vi "THz Time(SR830_VC_PSD_MCS)_TA_170401.vi"(4 "Lockin Address":string="12") -> ()   [LabVIEW 2010]
panel:
  in  "?":bool
  out "Current Round":i32=160
  out "Current Gap (um)":u32=100
  out "error out 2":errorcluster
  in  "Initial Gap (um)":u32=100
  in  "Number of Gap":u32=8
  in  "Number of Avg":u32=20
  in  "Gap Increase (um)":u32=25
  in  "Step Increase (um)":u32=1
  in  "error in (no error)":errorcluster
  in  "MCS System Locator":string="usb:id:1441320285"
  in  "CONEX-PSD9 Instrument Key 2":string="CONEX-PSD (A6ULD73M)"
  in  "Exit Program":bool
  out "Y position":dbl=-5.0 format="%#.3p"
  out "X position":dbl=-5.0 format="%#.3p"
  out "Power meter":dbl format="%#.3p"
  in  "Launch server?":bool
  in  "Authorize?":bool=TRUE
  out "error out":errorcluster
  out "Position 2":dbl[](array[numeric])=[2.395] format="%.6f"
  in  "error in":errorcluster
  out "Running":bool caption="Mercury_GCS_Configuration_Setup.vi is running"
  out "Conn. Axis":string[](array[string])=["1"]
  out "Identification":string="(c)2013 Physik Instrumente(PI) Karlsruhe, C-863.11,0,1.3.0.7"
  in  "SaveFile name":string="t"
  in  "Interdelay (ms)":dbl=10.0
  in  "pre delay (ms)":dbl=100.0
  out "Lock-in Y-Channel":dbl=-7.0941e-11 format="%#.3p"
  out "Lock-in X-Channel":dbl=5.62071e-10 format="%#.3p"
  out "THz Time-domain Signal Wave":cluster{"x-axis":sgl[], "y-axis":dbl[]}(graph)={"x-axis"=[3.4, 3.395, 3.39, 3.385, 3.38, 3.375, 3.3700001, 3.365, 3.3600001, 3.355, 3.3500001, 3.345, 3.3400002, 3.335, 3.3300002, 3.325, 3.3200002, 3.315, 3.3100002, 3.305, 3.3000002, 3.295, 3.2900002, 3.285, 3.2800002, 3.275, 3.27, 3.265, 3.26, 3.255, 3.25, 3.2450001, 3.24, 3.2350001, 3.23, 3.2250001, 3.22, 3.2150002, 3.21, 3.2050002, 3.2, 3.1950002, 3.19, 3.1850002, 3.18, 3.1750002, 3.17, 3.1650002, 3.16, 3.1550002, 3.15, 3.1450002, 3.14, 3.135, 3.13, 3.125, 3.1200001, 3.115, 3.1100001, 3.105, 3.1000001, 3.095, 3.0900002, 3.085, 3.0800002, 3.075, 3.0700002, 3.065, 3.0600002, 3.055, 3.0500002, 3.045, 3.0400002, 3.035, 3.0300002, 3.025, 3.0200002, 3.015, 3.01, 3.005, 3.0, 2.9950001, 2.99, 2.9850001, 2.98, 2.9750001, 2.97, 2.9650002, 2.96, 2.9550002, 2.95, 2.9450002, 2.94, 2.9350002, 2.93, 2.9250002, 2.92, 2.9150002, 2.91, 2.9050002, 2.9, 2.8950002, 2.89, 2.885, 2.88, 2.875, 2.8700001, 2.865, 2.8600001, 2.855, 2.8500001, 2.845, 2.8400002, 2.835, 2.8300002, 2.825, 2.8200002, 2.815, 2.8100002, 2.805, 2.8000002, 2.795, 2.7900002, 2.785, 2.7800002, 2.775, 2.7700002, 2.765, 2.7600002, 2.755, 2.75, 2.7450001, 2.74, 2.7350001, 2.73, 2.7250001, 2.72, 2.7150002, 2.71, 2.7050002, 2.7, 2.6950002, 2.69, 2.6850002, 2.68, 2.6750002, 2.67, 2.6650002, 2.66, 2.6550002, 2.65, 2.6450002, 2.64, 2.6350002, 2.63, 2.625, 2.6200001, 2.615, 2.6100001, 2.605, 2.6000001, 2.595, 2.5900002, 2.585, 2.5800002, 2.575, 2.5700002, 2.565, 2.5600002, 2.555, 2.5500002, 2.545, 2.5400002, 2.535, 2.5300002, 2.525, 2.5200002, 2.515, 2.5100002, 2.505, 2.5, 2.4950001, 2.49, 2.4850001, 2.48, 2.4750001, 2.47, 2.4650002, 2.46, 2.4550002, 2.45, 2.4450002, 2.44, 2.4350002, 2.43, 2.4250002, 2.42, 2.4150002, 2.41, 2.4050002, 2.4, 2.3950002], "y-axis"=array[202 elements]}
  in  "Autosave Directory for Long-term Average Scan":path=path "D:/Soon/140901_delay_test/2_VC_delay_ESP_-2.35/1_VC_delay"
  in  "OK Button":bool
  out "Data Type":string="outp ? 1"
  in  "Enum":enum16{"X", "Y", "Abs"}(ring)
  in  "SCAN":bool
  in  "Short term \nAverage#":i8=2
  in  "Step":sgl=0.005 min=0 max=10000 format="%.3f"
  in  "End Postion":sgl=2.4 min=-400 max=400 format="%#.3f"
  in  "Start Position":sgl=3.4 min=-400 max=400 format="%#.3f"
  # "THz Experiment"
  # "``"
  # "Input Data"
  # "Auto-offset"
  # "Point Avg"
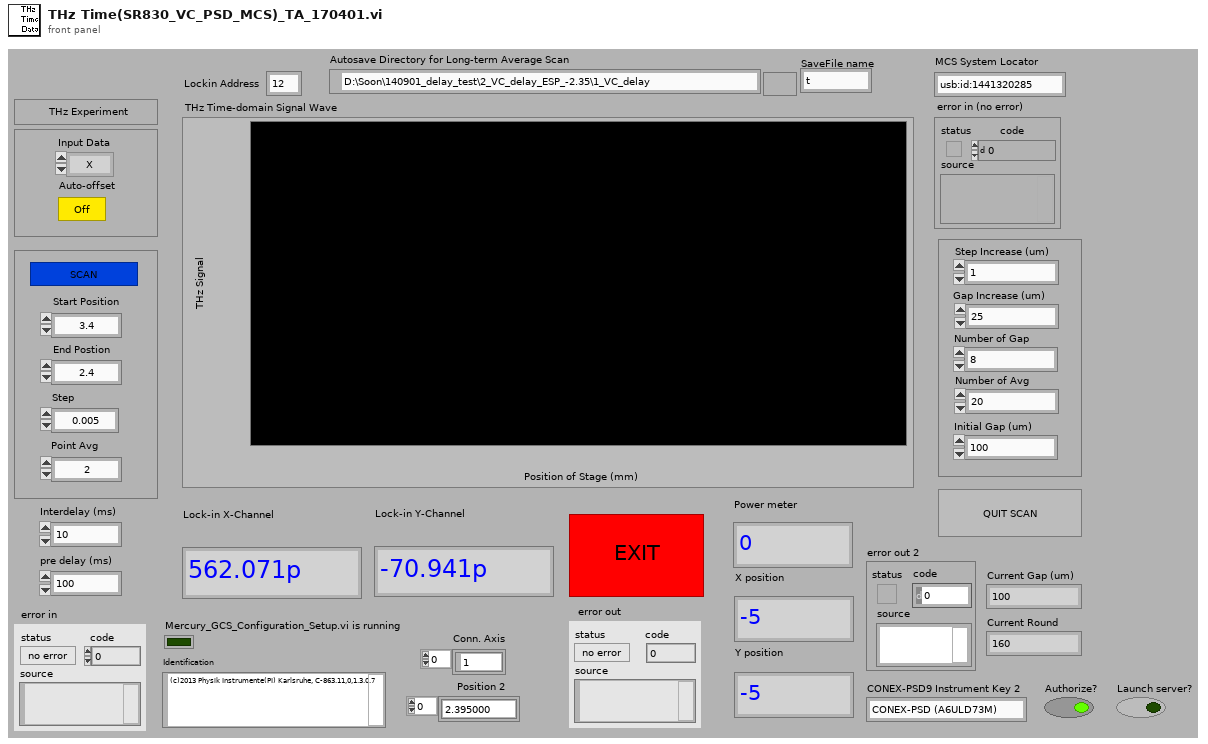
[diagram p1: front panel]
types:
  T1 = cluster{"System no.":i32, "error out":errorcluster}
  T2 = cluster{"ConexPSD Reference":refnum<k24>, "error out":errorcluster, "Component ID":i32}
  T3 = cluster{"System Index Out":u32, "error out":errorcluster}
  T4 = cluster{"Step Number":i32, "Step":sgl, "Start Position":sgl, "Time-out":i32, "Lockin Address":string, "Short term \nAverage#":i8, "System no.":i32, "error out":errorcluster, "Value":string, "pre delay (ms)":dbl, "Interdelay (ms)":dbl, "Autosave Directory for Long-term Average Scan":path, cluster{"ConexPSD Reference":refnum<k24>, "error out":errorcluster, "Component ID":i32}}
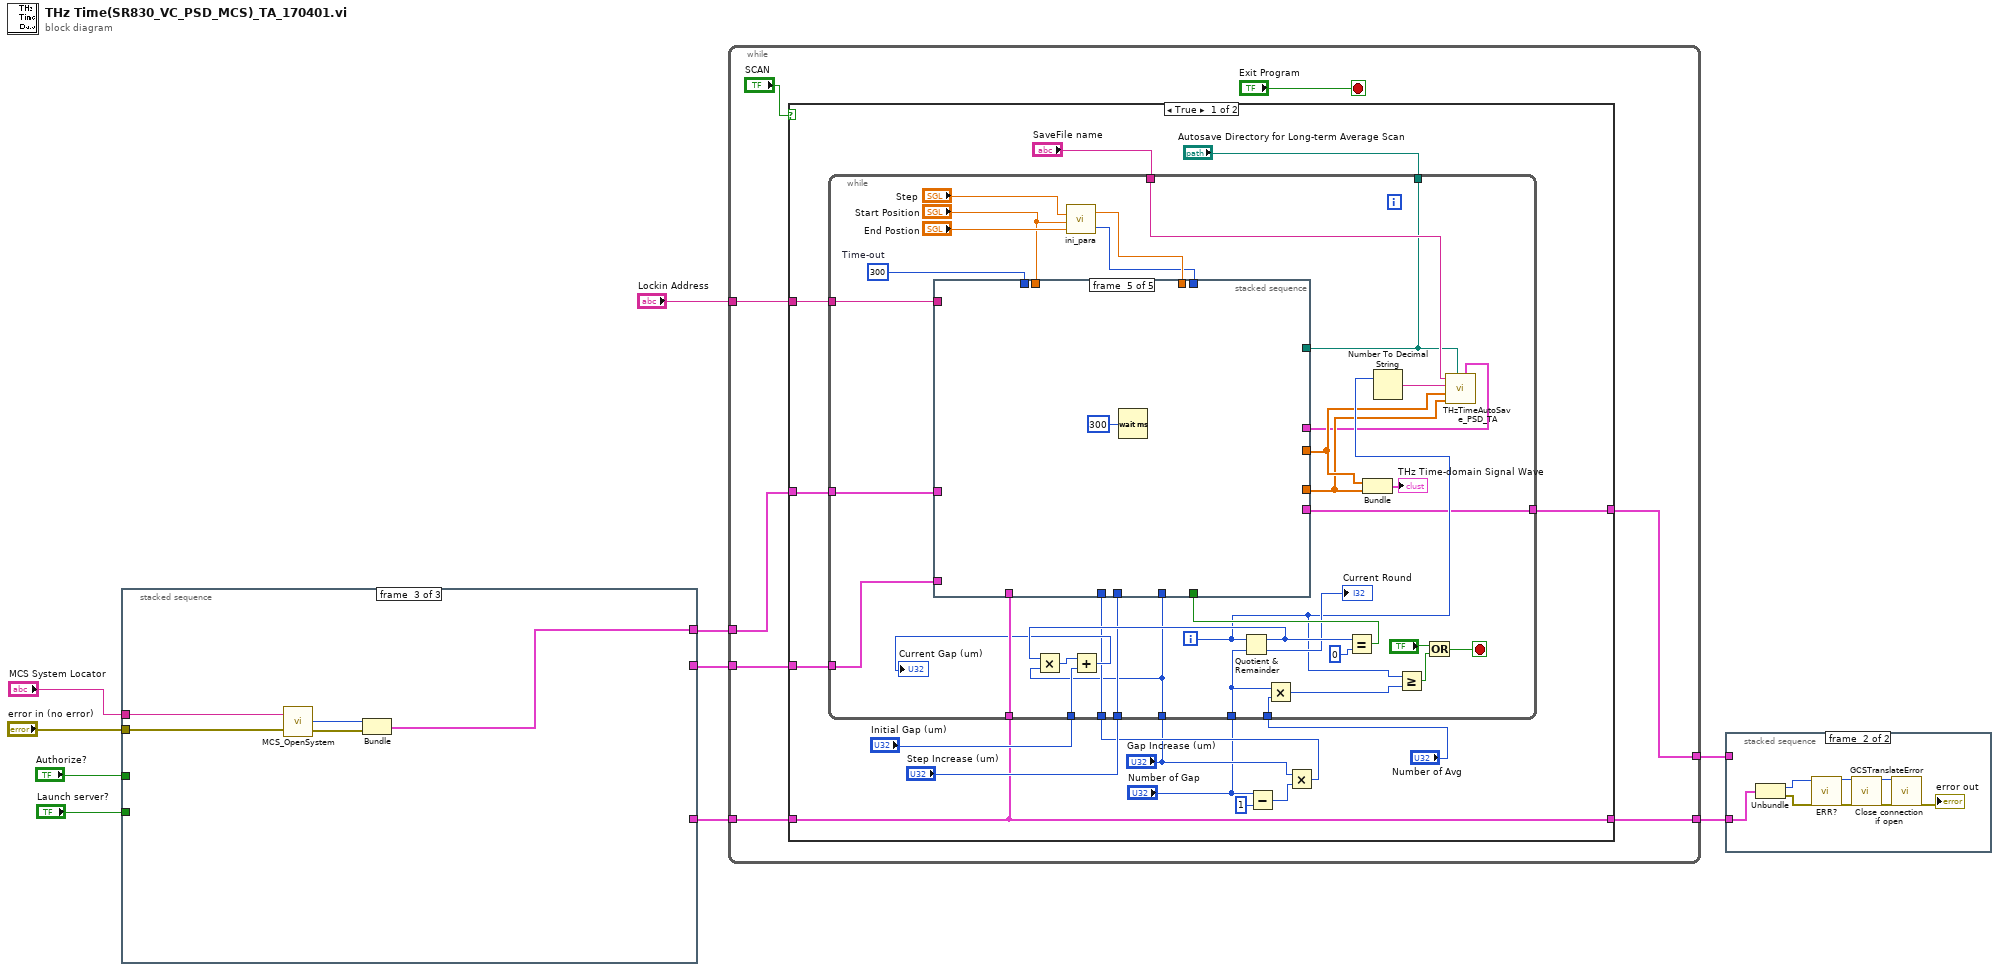
[diagram p0: block diagram]
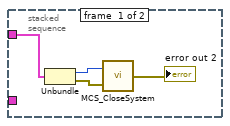
[diagram p2: hidden frame]
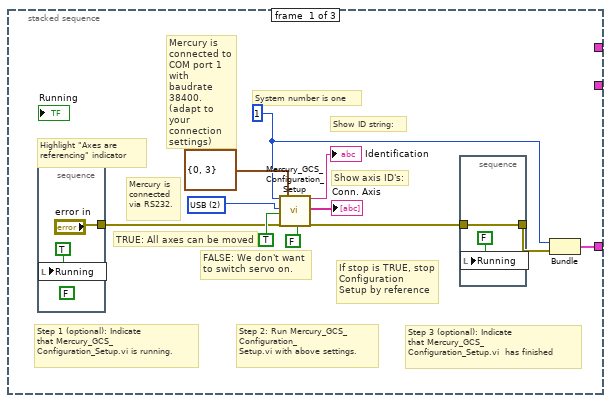
[diagram p3: hidden frame]
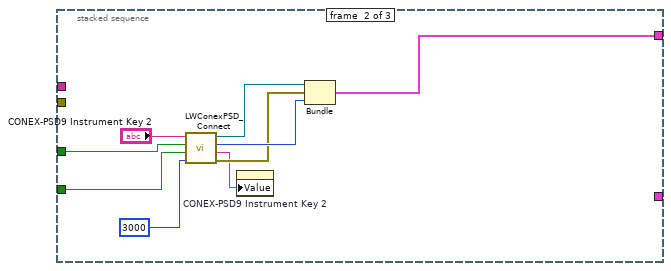
[diagram p4: hidden frame]
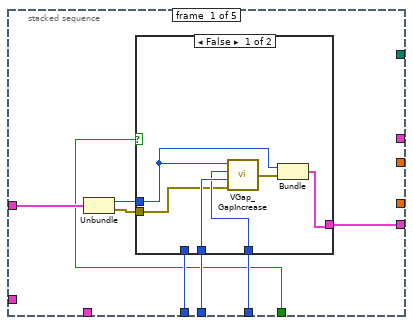
[diagram p5: hidden frame]
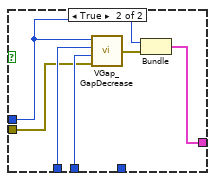
[diagram p6: hidden frame]
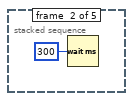
[diagram p7: hidden frame]
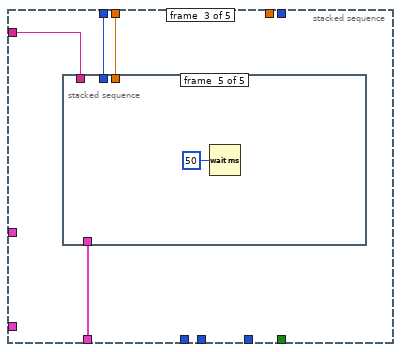
[diagram p8: hidden frame]
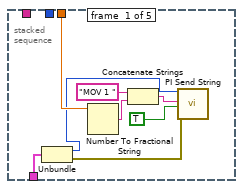
[diagram p9: hidden frame]
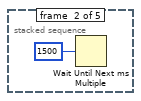
[diagram p10: hidden frame]
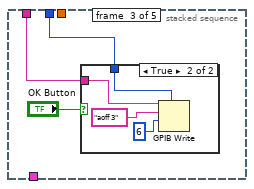
[diagram p11: hidden frame]
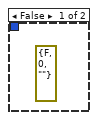
[diagram p12: hidden frame]
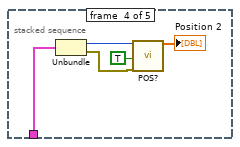
[diagram p13: hidden frame]
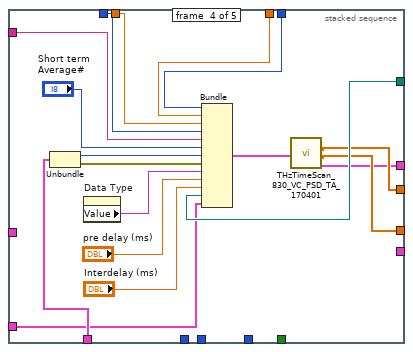
[diagram p14: hidden frame]
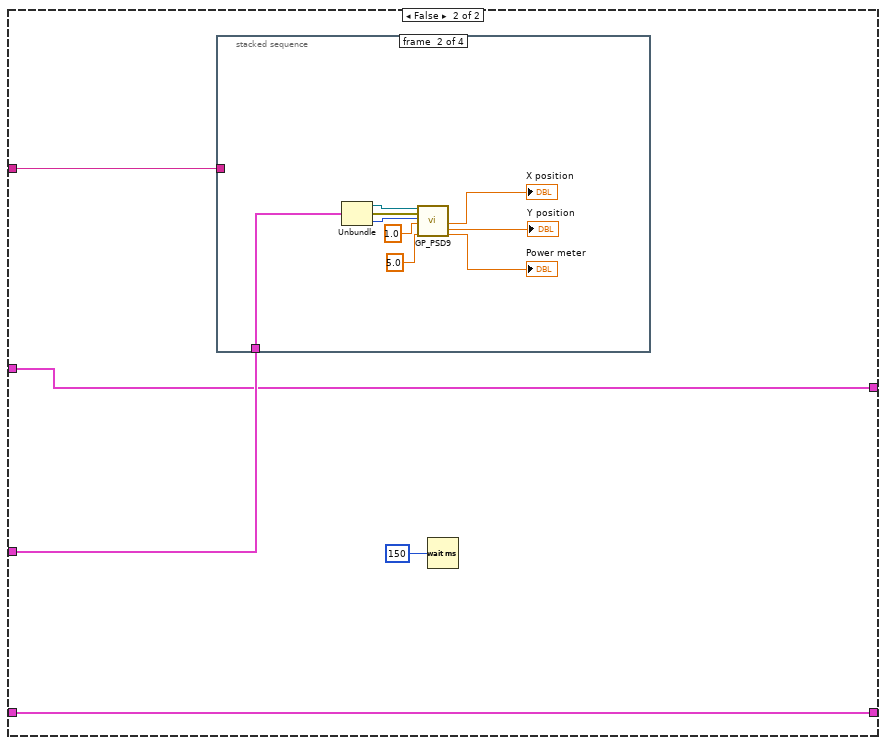
[diagram p15: hidden frame]
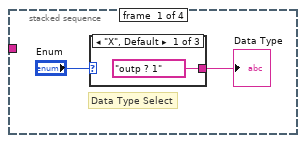
[diagram p16: hidden frame]
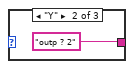
[diagram p17: hidden frame]
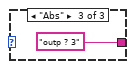
[diagram p18: hidden frame]
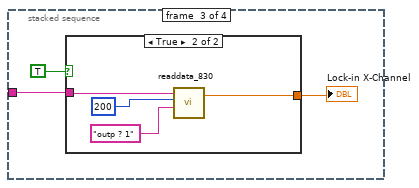
[diagram p19: hidden frame]
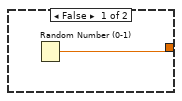
[diagram p20: hidden frame]
diagram:
  n1 = stacked-sequence {
    tunnel: "Authorize?" -> [_ w29 _]
    tunnel: "Launch server?" -> [_ w28 _]
    tunnel: [_ w26 _] -> w7
    tunnel: "MCS System Locator" -> [_ _ w37]
    tunnel: "error in (no error)" -> [_ _ w36]
    tunnel: [_ _ w35] -> w4
    tunnel: [w11 _ _] -> w3
    frame #0 {
      w14 = u16 2 items=["RS232", "RS232 DaisyChain", "USB", "USB_DaisyChain"] ("Interface")
      w12 = 1 ("System no.")
      # "Mercury is\nconnected\nvia RS232."
      # "If stop is TRUE, stop \nConfiguration\nSetup by reference"
      # "Mercury is\nconnected to\nCOM port 1\nwith baudrate\n38400.\n(adapt to your\nconnection\nsettings)"
      # "Step 3 (optional): Indicate\nthat Mercury_GCS_\nConfiguration_Setup.vi  has finished"
      # "Step 2: Run Mercury_GCS_\nConfiguration_\nSetup.vi with above settings."
      # "Step 1 (optional): Indicate\nthat Mercury_GCS_\nConfiguration_Setup.vi is running."
      # "Highlight \"Axes are\nreferencing\" indicator"
      # "Show axis ID's:"
      # "Show ID string:"
      # "FALSE: We don't want\nto switch servo on."
      # "TRUE: All axes can be moved"
      # "System number is one"
      n2 = stacked-sequence {
        tunnel: ["error in"] -> w17
        frame #0 {
          (unwired) FALSE ("stop")
          n3 = local write "Running"(TRUE ("Running")) -> ()
        }
      }
      n4 = call "Mercury_GCS_Configuration_Setup.vi"("System no."=w12, "Interface"=w14, "All axes?"=TRUE, "error in"=w17, "RS232 settings"=cluster{"RS232 Portnumber":i32, "Baudrate":u16} {"RS232 Portnumber"=0, "Baudrate"=3}, "Switch servo on?"=FALSE ("Use dialog to define\nconnected stages?")) -> ("Identification"=→"Identification":string, "Conn. \nAxes"=→"Conn. Axis":string[], "error out"=w18:errorcluster)  [unwired: 7 in, 4 out]
      n5 = stacked-sequence {
        tunnel: w18 -> [w25]
        tunnel: [w25] -> w13
        frame #0 {
          n6 = local write "Running"(FALSE ("Running")) -> ()
        }
      }
      n7 = Bundle("System no."=w12, "error out"=w13) -> (w11:T1)  [unwired: 1 in]
    }
    frame #1 {
      n8 = call "LWConexPSD_Connect.vi"("DiscoverTimeout (10000 msec)"=3000, "Launch server? (True)"=w28, "Authorize? (True)"=w29, "Instrument Key"="CONEX-PSD9 Instrument Key 2") -> ("error out"=w32:errorcluster, "Instrument Key out"=w31:string, "Component ID"=w33:i32, "ConexPSD Reference"=w27:refnum<k24>)
      n9 = property on="CONEX-PSD9 Instrument Key 2" class="Str"("Value"=w31) -> ()  [unwired: 2 in, 2 out]
      n10 = Bundle("ConexPSD Reference"=w27, "error out"=w32, "Component ID"=w33) -> (w26:T2)  [unwired: 1 in]
    }
    frame #2 {
      n11 = call "MCS_OpenSystem.vi"("error in (no error)"=w36, "MCS System Locator"=w37) -> ("error out"=w38:errorcluster, "System Index Out"=w39:u32)
      n12 = Bundle("System Index Out"=w39, "error out"=w38) -> (w35:T3)  [unwired: 1 in]
    }
  }
  n13 = while {
    tunnel: "Lockin Address" -> [w46]
    tunnel: w7 -> [w44]
    tunnel: w4 -> [w43]
    tunnel: w3 -> [w42]
    tunnel: [w41] -> w2
    tunnel: [w40] -> w1
    stop <- "Exit Program" stop-if-true
    n14 = case shown="True" "SCAN" {
      tunnel: w46 -> [w62 w167]
      tunnel: [w55 w165] -> w41
      tunnel: w44 -> [w49 w166]
      tunnel: w43 -> [w59 w164]
      tunnel: w42 -> [w55 w165]
      tunnel: [w48 w164] -> w40
      frame True {
        n15 = Subtract(x="Number of Gap", y=u32 1) -> (x-y=w53:u32)
        n16 = Multiply(x="Gap Increase (um)", y=w53) -> (x*y=w52:u32)
        n17 = while {
          tunnel: w62 -> [w97]
          tunnel: w55 -> [w96]
          tunnel: "SaveFile name" -> [w68]
          tunnel: "Autosave Directory for Long-term Average Scan" -> [w67]
          tunnel: w59 -> [w95]
          tunnel: "Initial Gap (um)" -> [w80]
          tunnel: "Step Increase (um)" -> [w77]
          tunnel: "Number of Avg" -> [w79]
          tunnel: w52 -> [w78]
          tunnel: "Gap Increase (um)" -> [w76]
          tunnel: "Number of Gap" -> [w75]
          tunnel: w49 -> [w66]
          tunnel: [w63] -> w48
          i -> [w71]
          stop <- w64 stop-if-true
          w94 = 300  # Time-out
          n18 = call "ini_para.vi"("End Position"="End Postion", "Start Position"="Start Position", "Step"="Step") -> ("Step Number"=w88:i32, "Step"=w89:sgl)
          n19 = Quotient & Remainder(x=w71, y=w75) -> (x-y*floor(x/y)=w86:u32, floor(x/y)=→"Current Round":u32)
          n20 = Multiply(x=w86, y=w76) -> (x*y=w85:u32)
          n21 = Add(x=w85, y=w80) -> (x+y=→"Current Gap (um)":u32)
          n22 = Multiply(x=w75, y=w79) -> (x*y=w82:u32)
          n23 = Equal?(x=w86, y=u32 0) -> (x = y?=w74:bool)
          n24 = stacked-sequence {
            tunnel: w94 -> [_ _ w122 w161 _]
            tunnel: "Start Position" -> [_ _ w121 w153 _]
            tunnel: w89 -> [_ _ _ w154 _]
            tunnel: w88 -> [_ _ _ w162 _]
            tunnel: [_ _ _ w146 _] -> w70
            tunnel: [_ _ _ w147 _] -> w69
            tunnel: w67 -> [_ _ _ w156 _]
            tunnel: w97 -> [_ _ w120 w155 _]
            tunnel: w96 -> [_ _ w119 w152 _]
            tunnel: w95 -> [w103 _ _ _ _]
            tunnel: w78 -> [w102 _ _ _ _]
            tunnel: w77 -> [w101 _ _ _ _]
            tunnel: w76 -> [w100 _ _ _ _]
            tunnel: w74 -> [w99 _ _ _ _]
            tunnel: w66 -> [_ _ _ w148 _]
            tunnel: [_ _ _ w145 _] -> w65
            tunnel: [w98 _ _ _ _] -> w63
            frame #0 {
              n25 = Unbundle(w103) -> ("System Index Out"=w104:u32, "error out"=w105:errorcluster)
              n26 = case shown="False" w99 {
                tunnel: w102 -> [_ w117]
                tunnel: w101 -> [w111 w116]
                tunnel: w100 -> [w110 _]
                tunnel: w104 -> [w107 w113]
                tunnel: w105 -> [w109 w115]
                tunnel: [w106 w112] -> w98
                frame False {
                  n27 = call "VGap_GapIncrease.vi"("error in (no error)"=w109, "Step Increase (um)"=w111, "Gap Increase (um)"=w110, "System Index In"=w107) -> ("error out"=w108:errorcluster)
                  n28 = Bundle("System Index Out"=w107, "error out"=w108) -> (w106:T3)  [unwired: 1 in]
                }
                frame True {
                  n29 = call "VGap_GapDecrease.vi"("error in (no error)"=w115, "Step Decrease (um)"=w116, "Gap Decrease (um)"=w117, "System Index In"=w113) -> ("error out"=w114:errorcluster)
                  n30 = Bundle("System Index Out"=w113, "error out"=w114) -> (w112:T3)  [unwired: 1 in]
                }
              }
            }
            frame #1 {
              n31 = Wait (ms)(milliseconds to wait=u32 300) -> ()  [unwired: 1 out]
            }
            frame #2 {
              n32 = stacked-sequence {
                tunnel: w122 -> [_ _ w133 _ _]
                tunnel: w121 -> [w126 _ _ _ _]
                tunnel: w120 -> [_ _ w132 _ _]
                tunnel: w119 -> [w125 _ _ w141 _]
                frame #0 {
                  n33 = Unbundle(w125) -> ("System no."=w123:i32, "error out"=w124:errorcluster)
                  n34 = Number To Fractional String(number=w126) -> (F-format string=w127:string)  [unwired: 3 in]
                  n35 = Concatenate Strings("MOV 1 ", w127) -> (w130:string)
                  n36 = call "PI Send String.vi"("System no."=w123, "String to send"=w130, "Attach termination char.?"=TRUE ("Attach Linefeed?"), "error in"=w124) -> ()  [unwired: 15 in, 1 out]
                }
                frame #1 {
                  n37 = Wait Until Next ms Multiple(millisecond multiple=1500) -> ()  [unwired: 1 out]
                }
                frame #2 {
                  n38 = case shown="True" "OK Button" {
                    tunnel: w133 -> [_ w137]
                    tunnel: w132 -> [_ w135]
                    frame False {
                      (unwired) errorcluster {"status"=FALSE, "code"=0, "source"=""} ("error in")
                    }
                    frame True {
                      n39 = GPIB Write(0:w135, 1:"aoff 3" ("data"), 2:i16 6 ("mode (0)"), 4:w137) -> ()  [unwired: 1 in, 2 out]
                    }
                  }
                }
                frame #3 {
                  n40 = Unbundle(w141) -> ("System no."=w140:i32, "error out"=w139:errorcluster)
                  n41 = call "POS?.vi"("System no."=w140, "All axes?"=TRUE, "error in"=w139) -> ("Position"=→"Position 2":dbl[])  [unwired: 15 in, 1 out]
                }
                frame #4 {
                  n42 = Wait (ms)(milliseconds to wait=u32 50) -> ()  [unwired: 1 out]
                }
              }
            }
            frame #3 {
              n43 = Unbundle(w152) -> ("System no."=w151:i32, "error out"=w150:errorcluster)
              n44 = property on="Data Type" class="Str"() -> ("Value"=w159:string)  [unwired: 2 in, 2 out]
              n45 = Bundle("Step Number"=w162, "Step"=w154, "Start Position"=w153, "Time-out"=w161, "Lockin Address"=w155, "Short term \nAverage#"="Short term \nAverage#", "System no."=w151, "error out"=w150, "Value"=w159, "pre delay (ms)"="pre delay (ms)", "Interdelay (ms)"="Interdelay (ms)", "Autosave Directory for Long-term Average Scan"=w156, w148) -> (w149:T4)  [unwired: 1 in]
              n46 = call "THzTimeScan_830_VC_PSD_TA_170401.vi"("input"=w149) -> ("x-axis"=w146:sgl[], "y-axis"=w147:dbl[], "ext. out"=w145:cluster{dbl[], dbl[], dbl[], dbl[], string[]})  [unwired: 1 out]
            }
            frame #4 {
              n47 = Wait (ms)(milliseconds to wait=u32 300) -> ()  [unwired: 1 out]
            }
          }
          n48 = Bundle("x-axis"=w70, "y-axis"=w69) -> (→"THz Time-domain Signal Wave":cluster{"x-axis":sgl[], "y-axis":dbl[]})  [unwired: 1 in]
          n49 = Number To Decimal String(number=w71) -> (decimal integer string=w72:string)  [unwired: 1 in]
          n50 = Greater Or Equal?(x=w71, y=w82) -> (x >= y?=w83:bool)
          n51 = Or(x="?", y=w83) -> (x .or. y?=w64:bool)
          n52 = call "THzTimeAutoSave_PSD_TA.vi"("ext. out"=w65, "Autosave Directory for Long-term Average Scan"=w67, "y-axis"=w69, "x-axis"=w70, "String"=w72, "SaveFile name"=w68) -> ()  [unwired: 4 in]
        }
      }
      frame False {
        n53 = stacked-sequence {
          tunnel: w167 -> [_ _ w183 w192]
          tunnel: w166 -> [_ w177 _ _]
          frame #0 {
            # "Data Type Select"
            n54 = case shown="\"X\", Default" "Enum" {
              tunnel: ["outp ? 1" "outp ? 2" "outp ? 3"] -> w170
              frame "X", Default {
              }
              frame "Y" {
              }
              frame "Abs" {
              }
            }
            "Data Type" <- w170
          }
          frame #1 {
            n55 = Unbundle(w177) -> ("ConexPSD Reference"=w182:refnum<k24>, "error out"=w181:errorcluster, "Component ID"=w180:i32)
            n56 = call "GP_PSD9.vi"("ConexPSD Reference"=w182, "error out"=w181, "Component ID"=w180, "Adress"=1.0 ("shot average"), "shot average"=5.0) -> ("PositionX"=→"X position":dbl, "PositionY"=→"Y position":dbl, "LaserPower"=→"Power meter":dbl)  [unwired: 8 in, 4 out]
          }
          frame #2 {
            n57 = case shown="True" TRUE {
              tunnel: [w186 w188] -> w185
              tunnel: w183 -> [_ w187]
              frame False {
                n58 = Random Number (0-1)() -> (number: 0 to 1=w186:dbl)
              }
              frame True {
                n59 = call "readdata_830.vi"("Command"="outp ? 1", "timeout"=200, "Lockin Address"=w187) -> ("Data"=w188:dbl)  [unwired: 1 in, 1 out]
              }
            }
            "Lock-in X-Channel" <- w185
          }
          frame #3 {
            n60 = case shown="True" TRUE {
              tunnel: w192 -> [_ w196]
              tunnel: [w194 w195] -> w191
              frame False {
                n61 = Random Number (0-1)() -> (number: 0 to 1=w194:dbl)
              }
              frame True {
                n62 = call "readdata_830.vi"("Command"="outp ? 2", "timeout"=200, "Lockin Address"=w196) -> ("Data"=w195:dbl)  [unwired: 1 in, 1 out]
              }
            }
            "Lock-in Y-Channel" <- w191
          }
        }
        n63 = Wait (ms)(milliseconds to wait=u32 150) -> ()  [unwired: 1 out]
      }
    }
  }
  n64 = stacked-sequence {
    tunnel: w1 -> [w199 _]
    tunnel: w2 -> [_ w205]
    frame #0 {
      n65 = Unbundle(w199) -> ("System Index Out"=w202:u32, "error out"=w201:errorcluster)
      n66 = call "MCS_CloseSystem.vi"("error in (no error)"=w201, "System Index In"=w202) -> ("error out"=→"error out 2":errorcluster)
    }
    frame #1 {
      n67 = Unbundle(w205) -> ("System no."=w204:i32, "error out"=w203:errorcluster)
      n68 = call "ERR?.vi"("error in"=w203) -> ("error out"=w207:errorcluster)  [unwired: 17 in, 1 out]
      n69 = call "GCSTranslateError.vi"("error in"=w207) -> ("error out"=w208:errorcluster)  [unwired: 16 in, 2 out]
      n70 = call "Close connection if open.vi"("System no."=w204, "error in"=w208) -> ("error out"=→"error out":errorcluster)  [unwired: 16 in, 1 out]
    }
  }
